vi "KeywordReadBinary.vi"(0 "Service":string, 2 "Keyword":string, 4 "Crate":string, 9 "error in (no error)":errorcluster) -> (3 "Value":string, 6 "error out":errorcluster)   [LabVIEW 2009]
uses:
  Controls/KeywordCommand.ctl
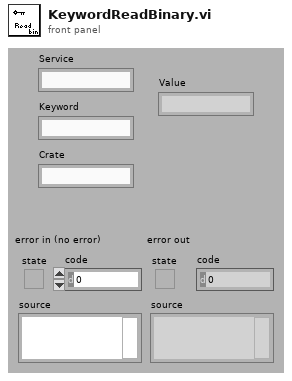
[diagram p1: front panel]
types:
  T1 = typedef "KeywordCommand.ctl" = cluster{"Command":enum16{"READ", "READBINARY", "WRITE", "QUIT"}, "Service":string, "Keyword":string, "Value":string, "done?":refnum<k4>}
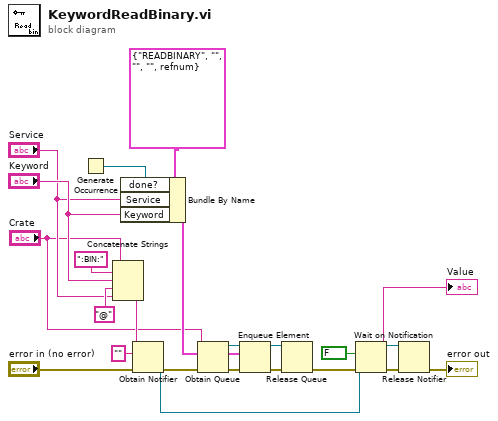
[diagram p0: block diagram]
diagram:
  n1 = Generate Occurrence() -> (w1:refnum<k4>)
  n2 = Concatenate Strings("Crate", ":BIN:" ("chaîne"), "Keyword", "@" ("chaîne"), "Service") -> (w11:string)
  n3 = Bundle By Name(cluster=T1 {"Command"=enum."READBINARY", "Service"="", "Keyword"="", "Value"="", "done?"=refnum} ("KeywordCommand"), "done?"=w1, "Service"="Service", "Keyword"="Keyword") -> (w20:T1)
  n4 = Obtain Notifier(name (unnamed)=w11, notification data type="" ("Value"), error in (no error)="error in (no error)") -> (notifier out=w7:refnum<notifier>, error out=w12:errorcluster)  [unwired: 1 in, 1 out]
  n5 = Obtain Queue(name (unnamed)="Crate", element data type=w20, error in (no error)=w12) -> (queue out=w21:refnum<queue>, error out=w22:errorcluster)  [unwired: 2 in, 1 out]
  n6 = Enqueue Element(queue=w21, element=w20, error in (no error)=w22) -> (queue out=w18:refnum<queue>, error out=w19:errorcluster)  [unwired: 2 out]
  n7 = Release Queue(queue=w18, error in (no error)=w19) -> (error out=w9:errorcluster)  [unwired: 3 out]
  n8 = Wait on Notification(notifier=w7, ignore previous (F)=FALSE ("ignorer précédent (F)"), error in (no error)=w9) -> (notifier out=w6:refnum<notifier>, notification=→"Value":string, error out=w5:errorcluster)  [unwired: 2 out]
  n9 = Release Notifier(notifier=w6, error in (no error)=w5) -> (error out=→"error out":errorcluster)  [unwired: 3 out]
